vi "PTSequencer.dialog edit step.vi"(0 "Step List In":T4[](array[typedef]), 3 "i step":i32, 4 "new":bool, 5 "error in (no error)":errorcluster, 6 "read only":bool) -> (14 "Step List Out":T4[](array[typedef]), 16 "Step Out":T4, 18 "changed":bool, 19 "error out":errorcluster)   [LabVIEW 2014, in "PTSequencer.lvlib"]
uses:
  PTSequencer.lvlib
  _typedefs/method parameters/method parameters.xctl
  PTSequencer.step.ctl
  CSCore/CSSystem/CoreDefs/CoreDefs.rawDataType.ctl
  PTSequencer.DIM service condition.ctl
  _typedefs/X DIM conditions/X DIM conditions.xctl
  <vilib>/Utility/miscctls.llb/LVStringsAndValuesArrayTypeDef.ctl
  CSCore/CSSystem/CoreLib/CoreLib.byte array 2 string.vi
  CSCore/CSSystem/CoreLib/CoreLib.byte array 2 int.vi
  CSCore/CSSystem/CoreLib/CoreLib.byte array 2 int array.vi
  CSCore/CSSystem/CoreLib/CoreLib.byte array 2 short.vi
  CSCore/CSSystem/CoreLib/CoreLib.byte array 2 short array.vi
  CSCore/CSSystem/CoreLib/CoreLib.byte array 2 double.vi
  CSCore/CSSystem/CoreLib/CoreLib.byte array 2 double array.vi
  CSCore/CSSystem/CoreLib/CoreLib.byte array 2 float.vi
  CSCore/CSSystem/CoreLib/CoreLib.byte array 2 float array.vi
  _common/PTUtils/PTUtils.lvlib
  CSCore/CSSystem/CSSystemLib/CSSystemLib.lvlib
  CSCore/CSSystem/CoreLib/CoreLib.lvlib
panel:
  in  "Jump_failed":i32(ring) caption="if failed, jump to"
  in  "DIM Services ctl":T3
  in  "Delay":dbl caption="s"
  in  "delay":bool caption="use delay"
  out "Descriptors":string[](array[string])
  in  "DIM Services":T3(xcontrol) caption="DIM conditions"
  out "Errors":string
  in  "Step In":T4
  in  "Cancel":bool
  in  "Ok":bool
  out "subsequence":bool
  in  "Jump_passed":i32(ring) caption="if passed, jump to"
  in  "Failed":enum16{"Next", "Previous", "Repeat", "Jump"}(ring)
  in  "Passed":enum16{"Next", "Previous", "Repeat", "Jump"}(ring)
  in  "check":bool caption="use conditions"
  in  "Output Params":T5(xcontrol) caption="Output Parameters"
  in  "Input Params":T5(xcontrol) caption="Input Parameters"
  in  "Call Mode":enum16{"Simple DIM", "Synchronous"}(ring) caption="Call mode"
  in  "Method":u16(ring) items=["Ping", "GetDescriptors", "SetPdcInterval", "SetPdcPreset", "SetEvtPreset", "GetEvtStatus", "GetCNames", "GetIList", "Reset", "ReadData", "STOP", "Wait", "WakeupPeriodic", "GetVersionOfLibrary", "SetEvtPresetValue", "SetPdcPresetValue", "LoadProcess", "UnloadProcess", "RemoveAll", "ConnectProcess", "DisconnectProcess", "DisconnectAll", "GetClassNames", "GetObjectNames", "KillObject", "KillClass", "KillAllClasses", "SyncProcTable", "OpenFrontPanel", "RegisterProcess", "UnregisterProcess", "CreateObject", "DestroyObject"]
  in  "Object":u16(ring) items=["MainSystem\\Super", "MainSystem\\UserGOG", "MainSystem\\UserGOG_NotiObj", "OPCGatewayHV", "OPCGatewayLV", "PTScanner", "PT_CAEN_Gateway\\Super", "SimAFG"]
  in  "Description":string
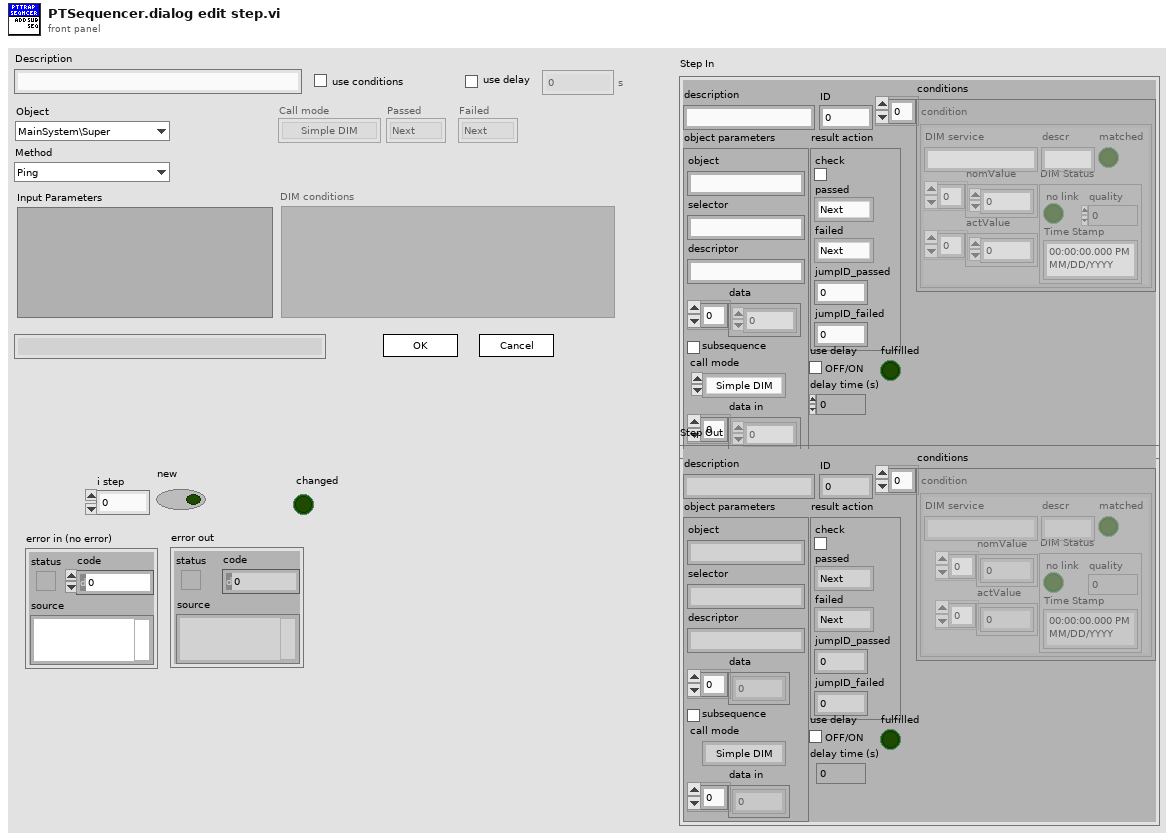
[diagram p1: front panel]
types:
  T1 = typedef "PTSequencer.lvlib/PTSequencer.DIM service condition.ctl" = cluster{"DIM service":string, "descr":string, "nomValue":T2, "actValue":T2, "matched":bool, "DIM Status":cluster{"no link":bool, "quality":i32, "Time Stamp":timestamp}}
  T2 = typedef "CoreDefs.rawDataType.ctl" = i8[]
  T3 = cluster{"DIM Services":string[], "data decsriptors":string[], "stop conditions":T1[]}
  T4 = typedef "PTSequencer.lvlib/PTSequencer.step.ctl" = cluster{"description":string, "object parameters":cluster{"object":string, "selector":string, "descriptor":string, "data":T2, "subsequence":bool, "call mode":enum16{"Simple DIM", "Synchronous"}, "data in":T2}, "result action":cluster{"check":bool, "passed":enum16{"Next", "Previous", "Repeat", "Jump"}, "failed":enum16{"Next", "Previous", "Repeat", "Jump"}, "jumpID_passed":i32, "jumpID_failed":i32}, "conditions":T1[], "fulfilled ":bool, "use delay":bool, "delay time (s)":dbl, "ID":i32}
  T5 = cluster{"Name":string, "Descr":string, "Value":string}[]
  T6 = enum8{"Enabled", "Disabled", "Disabled and Grayed Out"}
  T7 = typedef "LVStringsAndValuesArrayTypeDef.ctl" = cluster{"String":string, "Value":ext}[]
  T8 = cluster{"Name":string, "Descr":string, "Value":string}
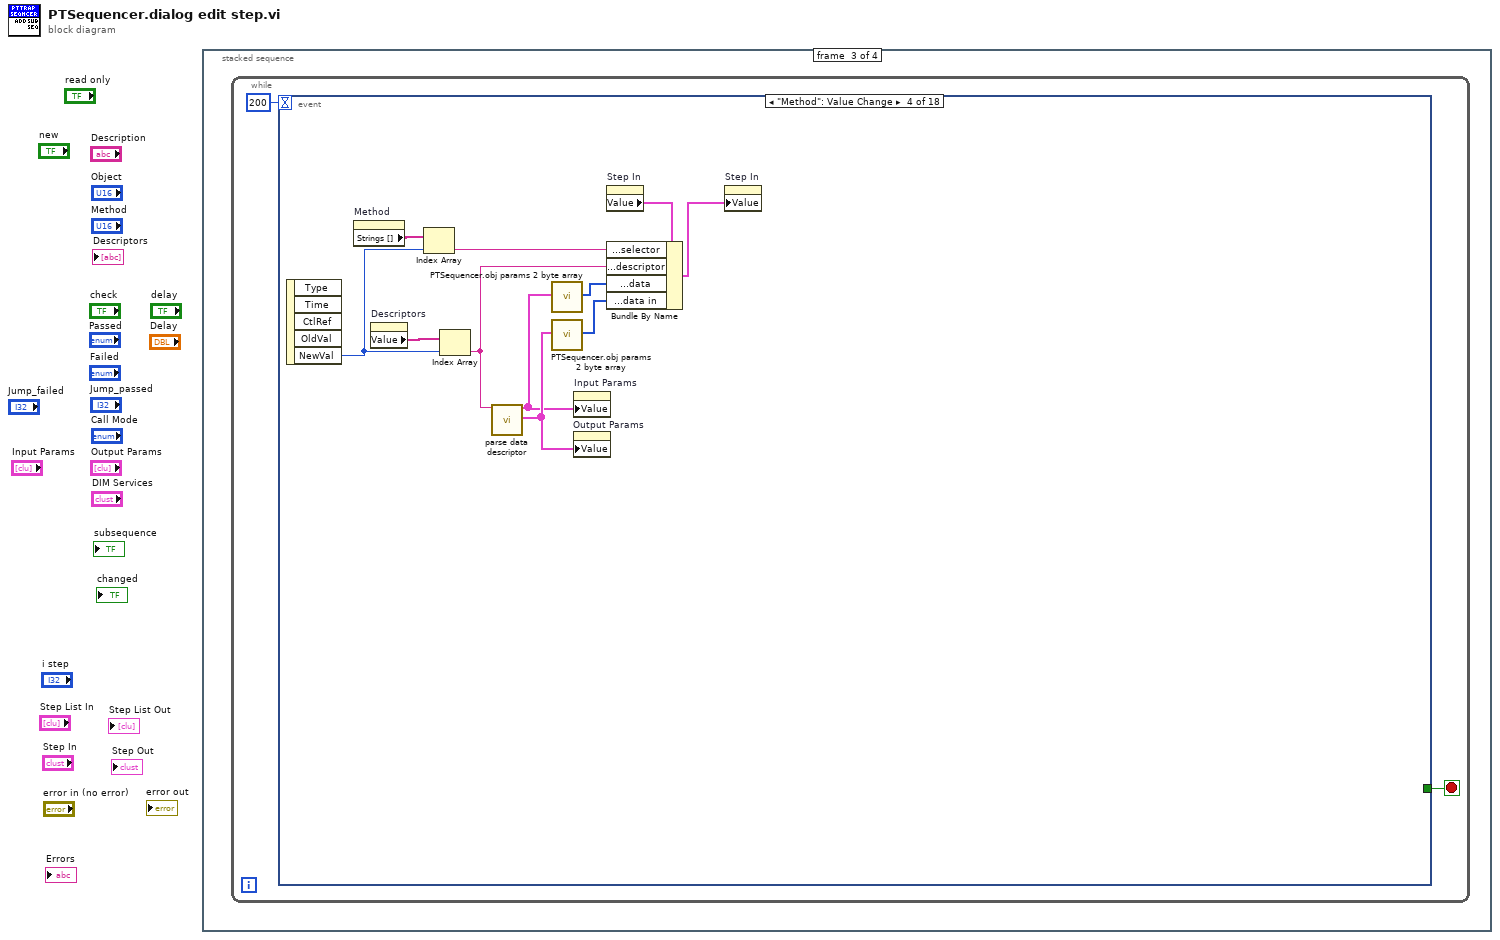
[diagram p0: block diagram]
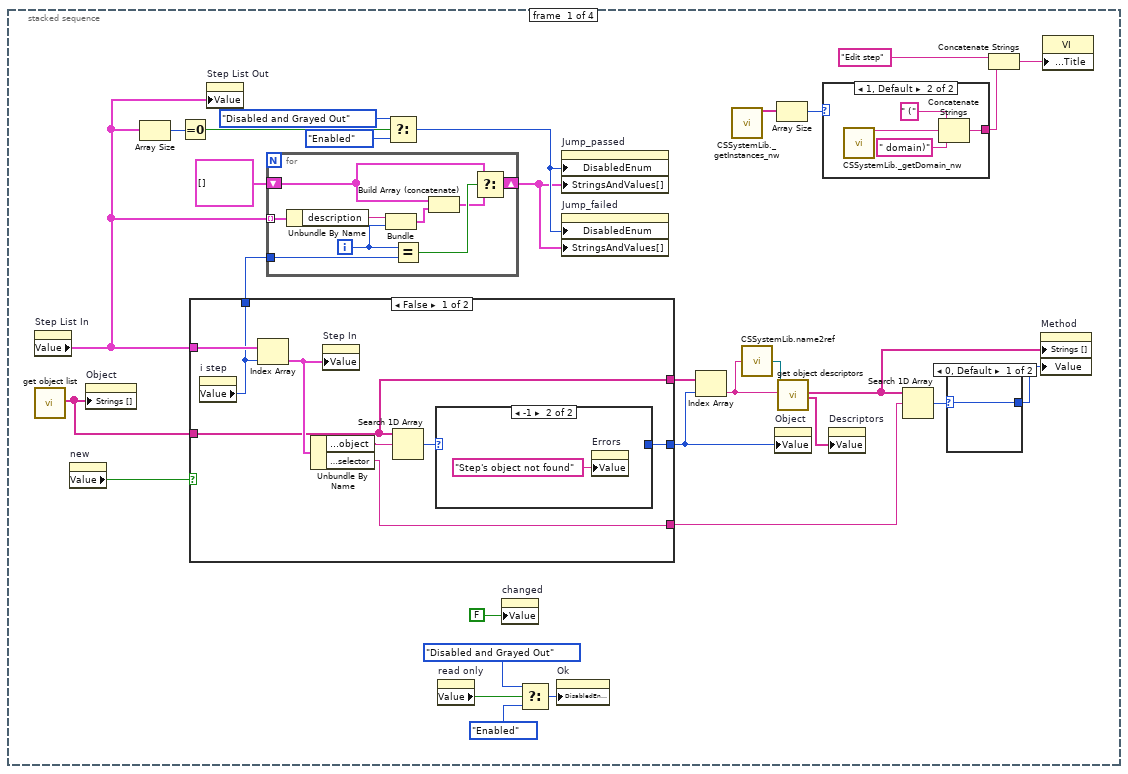
[diagram p2: hidden frame]
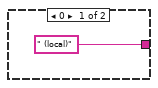
[diagram p3: hidden frame]
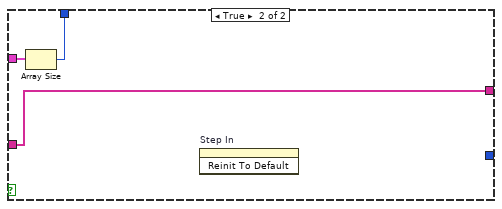
[diagram p6: hidden frame]
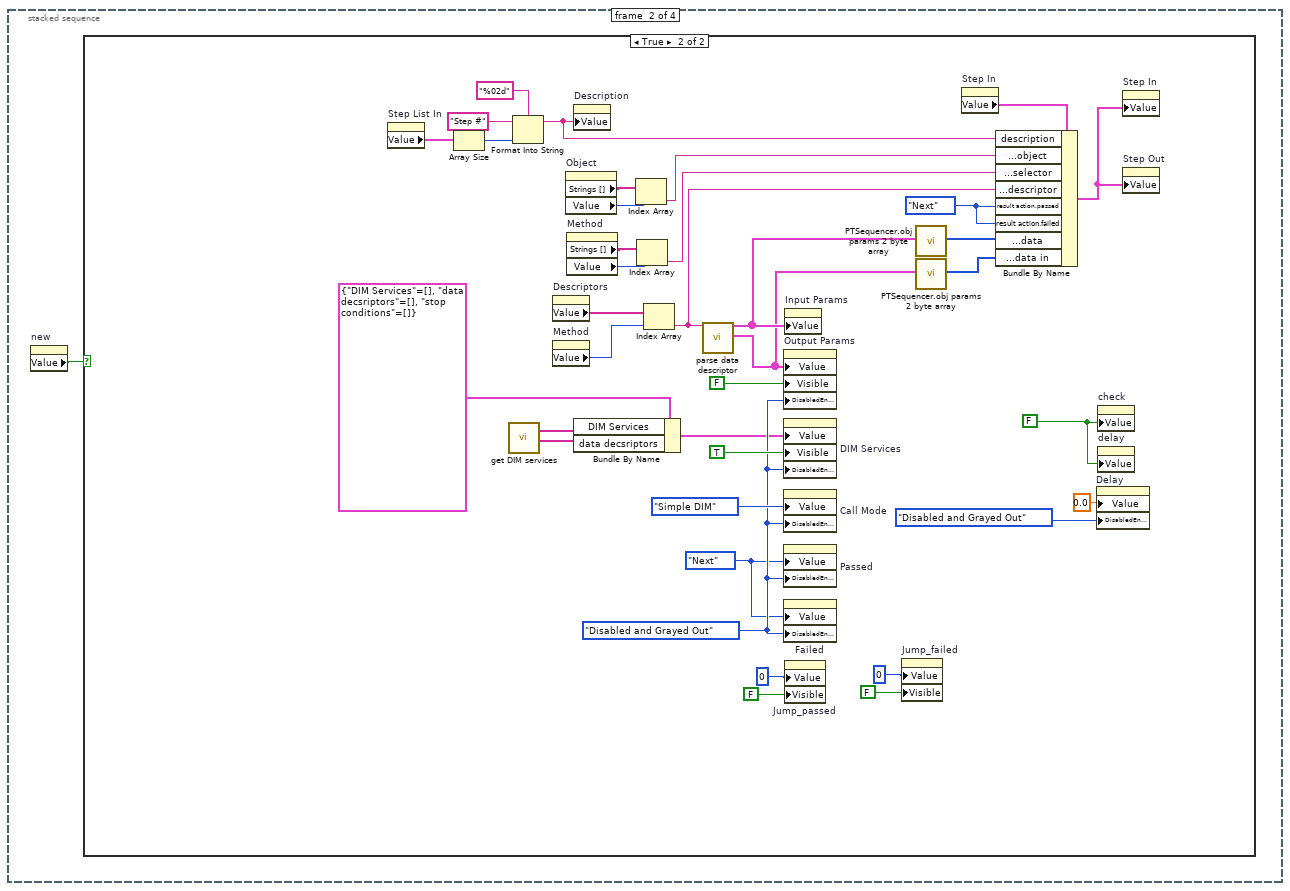
[diagram p7: hidden frame]
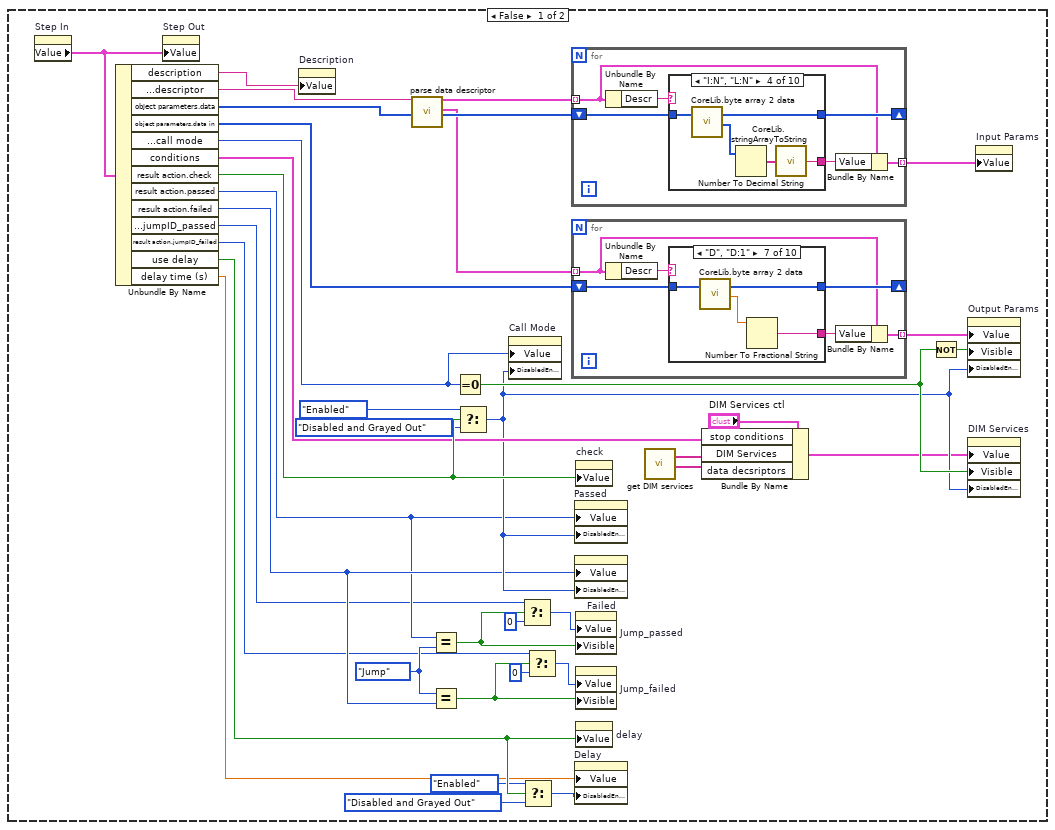
[diagram p8: hidden frame]
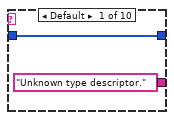
[diagram p9: hidden frame]
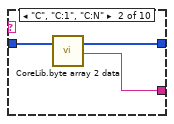
[diagram p10: hidden frame]
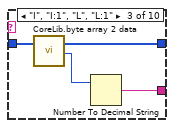
[diagram p11: hidden frame]
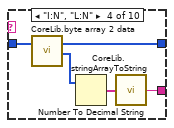
[diagram p12: hidden frame]
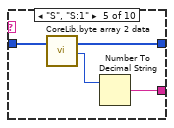
[diagram p13: hidden frame]
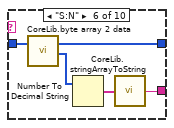
[diagram p14: hidden frame]
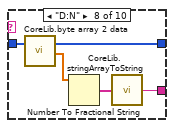
[diagram p15: hidden frame]
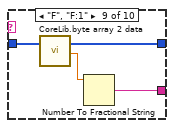
[diagram p16: hidden frame]
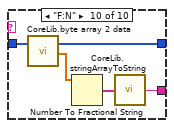
[diagram p17: hidden frame]
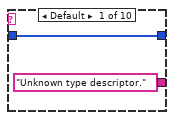
[diagram p18: hidden frame]
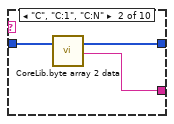
[diagram p19: hidden frame]
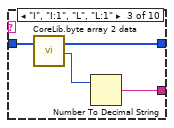
[diagram p20: hidden frame]
diagram:
  n1 = stacked-sequence {
    frame #0 {
      n2 = property on="Step List In" class="Arr (strict)"() -> ("Value"=w16:T4[])  [unwired: 2 in, 2 out]
      n3 = call "get object list.vi"() -> ("Objects"=w29:string[])  [unwired: 19 in]
      n4 = property on="new" class="Bool (strict)"() -> ("Value"=w30:bool)  [unwired: 2 in, 2 out]
      n5 = property on="Object" class="Ring (strict)"("Strings []"=w29) -> ()  [unwired: 2 in, 2 out]
      n6 = Array Size(array=w16) -> (size(s)=w15:i32)
      n7 = Equal To 0?(x=w15) -> (x = 0?=w14:bool)
      n8 = case shown="False" w30 {
        tunnel: w29 -> [w47 w58]
        tunnel: w16 -> [w50 w57]
        tunnel: [w49 w56] -> w27
        tunnel: [w48 _] -> w24
        tunnel: [w47 w58] -> w25
        tunnel: [w46 _] -> w22
        frame False {
          n9 = property on="i step" class="DigNum (strict)"() -> ("Value"=w49:i32)  [unwired: 2 in, 2 out]
          n10 = Index Array(array=w50, index=w49) -> (element=w53:T4)
          n11 = Unbundle By Name(w53) -> ("object parameters.object"=w52:string, "object parameters.selector"=w46:string)
          n12 = property on="Step In" class="Clust (strict)"("Value"=w53) -> ()  [unwired: 2 in, 2 out]
          n13 = Search 1D Array(1D array=w47, element=w52) -> (index of element=w51:i32)  [unwired: 1 in]
          n14 = case shown="-1" w51 {
            selector: w51 -> [w54 _]
            tunnel: [w54 _] -> w48
            frame 0, Default {
            }
            frame -1 {
              n15 = property on="Errors" class="Str"("Value"="Step's object not found") -> ()  [unwired: 2 in, 2 out]
            }
          }
        }
        frame True {
          n16 = Array Size(array=w57) -> (size(s)=w56:i32)
          n17 = invoke on="Step In" class="Clust (strict)" method="Reinit To Default"() -> ()  [unwired: 3 in, 3 out]
        }
      }
      n18 = property on="Step List Out" class="Arr (strict)"("Value"=w16) -> ()  [unwired: 2 in, 2 out]
      n19 = for {
        tunnel: w16 -> [w45] mode=indexing
        tunnel: w27 -> [w43]
        shift-right: [w37] -> w5
        shift-left: T7 [] ("Strings And Values []") -> [w38]
        i -> [w42]
        n20 = Unbundle By Name(w45) -> ("description"=w44:string)
        n21 = Bundle("description"=w44, w42) -> (w40:cluster{"description":string, i32})  [unwired: 1 in]
        n22 = Equal?(x=w42, y=w43) -> (x = y?=w41:bool)
        n23 = Build Array (concatenate)(w38, w40) -> (w39:T7)
        n24 = Select(t=w38, s=w41, f=w39) -> (s? t:f=w37:T7)
      }
      n25 = Select(t=T6."Disabled and Grayed Out" ("Disabled"), s=w14, f=T6."Enabled" ("Disabled")) -> (s? t:f=w6:T6)
      n26 = property on="read only" class="Bool (strict)"() -> ("Value"=w4:bool)  [unwired: 2 in, 2 out]
      n27 = property on="changed" class="Bool (strict)"("Value"=FALSE ("changed")) -> ()  [unwired: 2 in, 2 out]
      n28 = Select(t=T6."Disabled and Grayed Out" ("Disabled"), s=w4, f=T6."Enabled" ("Disabled")) -> (s? t:f=w3:T6)
      n29 = property on="Ok" class="Bool"("DisabledEnum"=w3) -> ()  [unwired: 2 in, 2 out]
      n30 = property on="Jump_passed" class="Ring (strict)"("DisabledEnum"=w6, "StringsAndValues[]"=w5) -> ()  [unwired: 2 in, 2 out]
      n31 = property on="Jump_failed" class="Ring (strict)"("DisabledEnum"=w6, "StringsAndValues[]"=w5) -> ()  [unwired: 2 in, 2 out]
      n32 = Index Array(array=w25, index=w24) -> (element=w23:string)
      n33 = call "CSSystemLib._getInstances_nw.vi"() -> ("i list"=w10:string[])  [unwired: 18 in, 1 out]
      n34 = call "CSSystemLib.name2ref.vi"("name"=w23) -> ("obj refnum"=w26:refnum<vi>)
      n35 = property on="Object" class="Ring (strict)"("Value"=w24) -> ()  [unwired: 2 in, 2 out]
      n36 = Array Size(array=w10) -> (size(s)=w11:i32)
      n37 = call "get object descriptors.vi"("i ref in"=w26, "Object"=w23) -> ("selectors"=w21:string[], "Descriptors"=w18:string[])  [unwired: 14 in, 2 out]
      n38 = case shown="1, Default" w11 {
        tunnel: [" (local)" w32] -> w8
        frame 0 {
        }
        frame 1, Default {
          n39 = call "CSSystemLib._getDomain_nw.vi"() -> ("CSDomain"=w34:string)  [unwired: 18 in, 1 out]
          n40 = Concatenate Strings(" (", w34, " domain)") -> (w32:string)
        }
      }
      n41 = property on="Descriptors" class="Arr (strict)"("Value"=w18) -> ()  [unwired: 2 in, 2 out]
      n42 = Search 1D Array(1D array=w21, element=w22) -> (index of element=w20:i32)  [unwired: 1 in]
      n43 = case shown="0, Default" w20 {
        selector: w20 -> [w36 _]
        tunnel: [w36 _] -> w19
        frame 0, Default {
        }
        frame -1 {
        }
      }
      n44 = Concatenate Strings("Edit step", w8) -> (w7:string)
      n45 = property on="Method" class="Ring (strict)"("Strings []"=w21, "Value"=w19) -> ()  [unwired: 2 in, 2 out]
      n46 = property class="VI"("Front Panel Window:Title"=w7) -> ()  [unwired: 2 in, 2 out]
    }
    frame #1 {
      n47 = property on="new" class="Bool (strict)"() -> ("Value"=w59:bool)  [unwired: 2 in, 2 out]
      n48 = case shown="True" w59 {
        frame False {
          w67 = enum16{"Next", "Previous", "Repeat", "Jump"}."Jump" ("y")
          n49 = property on="Step In" class="Clust (strict)"() -> ("Value"=w74:T4)  [unwired: 2 in, 2 out]
          n50 = Unbundle By Name(w74) -> ("description"=w68:string, "object parameters.descriptor"=w96:string, "object parameters.data"=w95:T2, "object parameters.data in"=w94:T2, "object parameters.call mode"=w93:enum16{"Simple DIM", "Synchronous"}, "conditions"=w83:T1[], "result action.check"=w92:bool, "result action.passed"=w66:enum16{"Next", "Previous", "Repeat", "Jump"}, "result action.failed"=w79:enum16{"Next", "Previous", "Repeat", "Jump"}, "result action.jumpID_passed"=w60:i32, "result action.jumpID_failed"=w61:i32, "use delay"=w73:bool, "delay time (s)"=w70:dbl)
          n51 = property on="Step Out" class="Clust (strict)"("Value"=w74) -> ()  [unwired: 2 in, 2 out]
          n52 = property on="Description" class="Str"("Value"=w68) -> ()  [unwired: 2 in, 2 out]
          n53 = call "parse data descriptor.vi"("dataDescriptor"=w96) -> ("Input Parameters"=w91:T5, "Output Parameters"=w89:T5)  [unwired: 14 in, 3 out]
          n54 = Equal?(x=w66, y=w67) -> (x = y?=w63:bool)
          n55 = Equal?(x=w67, y=w79) -> (x = y?=w64:bool)
          n56 = Equal To 0?(x=w93) -> (x = 0?=w87:bool)
          n57 = Select(t=T6."Enabled" ("Disabled"), s=w92, f=T6."Disabled and Grayed Out" ("Disabled")) -> (s? t:f=w80:T6)
          n58 = property on="Call Mode" class="Enum (strict)"("Value"=w93, "DisabledEnum"=w80) -> ()  [unwired: 2 in, 2 out]
          n59 = Select(t=w60, s=w63, f=0) -> (s? t:f=w62:i32)
          n60 = Select(t=T6."Enabled" ("Disabled"), s=w73, f=T6."Disabled and Grayed Out") -> (s? t:f=w69:T6)
          n61 = Select(t=w61, s=w64, f=0) -> (s? t:f=w76:i32)
          n62 = for {
            tunnel: w91 -> [w146] mode=indexing
            shift-right: [w147] -> _
            shift-left: w95 -> [w148]
            tunnel: [w144] -> w90 mode=indexing
            n63 = Unbundle By Name(w146) -> ("Descr"=w149:string)
            n64 = case shown="\"I:N\", \"L:N\"" w149 {
              tunnel: w148 -> [w151 w154 w158 w163 w167 w172 w176 w181 w184 w188]
              tunnel: [w151 w153 w157 w159 w164 w171 w175 w180 w182 w186] -> w147
              tunnel: ["Unknown type descriptor." w152 w155 w160 w165 w168 w173 w177 w183 w187] -> w145
              frame Default {
              }
              frame "C", "C:1", "C:N" {
                n65 = call-poly "CoreLib.byte array 2 data.vi"("byteArray"=w154) -> ("byteArray out"=w153:T2, "string"=w152:string)  [unwired: 16 in, 1 out]
              }
              frame "I", "I:1", "L", "L:1" {
                n66 = call-poly "CoreLib.byte array 2 data.vi"("byteArray"=w158) -> ("byteArray out"=w157:T2, "i32"=w156:i32)  [unwired: 16 in, 1 out]
                n67 = Number To Decimal String(number=w156) -> (decimal integer string=w155:string)  [unwired: 1 in]
              }
              frame "I:N", "L:N" {
                n68 = call-poly "CoreLib.byte array 2 data.vi"("byteArray"=w163) -> ("byteArray out"=w159:T2, "[i32]"=w162:i32[])  [unwired: 16 in, 1 out]
                n69 = Number To Decimal String(number=w162) -> (decimal integer string=w161:string[])  [unwired: 1 in]
                n70 = call "CoreLib.stringArrayToString.vi"("Array"=w161) -> ("String"=w160:string)
              }
              frame "S", "S:1" {
                n71 = call-poly "CoreLib.byte array 2 data.vi"("byteArray"=w167) -> ("byteArray out"=w164:T2, "i16"=w166:i16)  [unwired: 16 in, 1 out]
                n72 = Number To Decimal String(number=w166) -> (decimal integer string=w165:string)  [unwired: 1 in]
              }
              frame "S:N" {
                n73 = call-poly "CoreLib.byte array 2 data.vi"("byteArray"=w172) -> ("byteArray out"=w171:T2, "[i16]"=w170:i16[])  [unwired: 16 in, 1 out]
                n74 = Number To Decimal String(number=w170) -> (decimal integer string=w169:string[])  [unwired: 1 in]
                n75 = call "CoreLib.stringArrayToString.vi"("Array"=w169) -> ("String"=w168:string)
              }
              frame "D", "D:1" {
                n76 = call-poly "CoreLib.byte array 2 data.vi"("byteArray"=w176) -> ("byteArray out"=w175:T2, "d64"=w174:dbl)  [unwired: 16 in, 1 out]
                n77 = Number To Fractional String(number=w174) -> (F-format string=w173:string)  [unwired: 3 in]
              }
              frame "D:N" {
                n78 = call-poly "CoreLib.byte array 2 data.vi"("byteArray"=w181) -> ("byteArray out"=w180:T2, "[d64]"=w179:dbl[])  [unwired: 16 in, 1 out]
                n79 = Number To Fractional String(number=w179) -> (F-format string=w178:string[])  [unwired: 3 in]
                n80 = call "CoreLib.stringArrayToString.vi"("Array"=w178) -> ("String"=w177:string)
              }
              frame "F", "F:1" {
                n81 = call-poly "CoreLib.byte array 2 data.vi"("byteArray"=w184) -> ("byteArray out"=w182:T2, "f32"=w185:sgl)  [unwired: 16 in, 1 out]
                n82 = Number To Fractional String(number=w185) -> (F-format string=w183:string)  [unwired: 3 in]
              }
              frame "F:N" {
                n83 = call-poly "CoreLib.byte array 2 data.vi"("byteArray"=w188) -> ("byteArray out"=w186:T2, "[f32]"=w190:sgl[])  [unwired: 16 in, 1 out]
                n84 = Number To Fractional String(number=w190) -> (F-format string=w189:string[])  [unwired: 3 in]
                n85 = call "CoreLib.stringArrayToString.vi"("Array"=w189) -> ("String"=w187:string)
              }
            }
            n86 = Bundle By Name(cluster=w146, "Value"=w145) -> (w144:T8)
          }
          n87 = for {
            tunnel: w89 -> [w99] mode=indexing
            shift-right: [w100] -> _
            shift-left: w94 -> [w101]
            tunnel: [w97] -> w88 mode=indexing
            n88 = Unbundle By Name(w99) -> ("Descr"=w102:string)
            n89 = case shown="\"D\", \"D:1\"" w102 {
              tunnel: w101 -> [w104 w107 w111 w116 w120 w125 w129 w134 w137 w141]
              tunnel: [w104 w106 w110 w112 w117 w124 w128 w133 w135 w139] -> w100
              tunnel: ["Unknown type descriptor." w105 w108 w113 w118 w121 w126 w130 w136 w140] -> w98
              frame Default {
              }
              frame "C", "C:1", "C:N" {
                n90 = call-poly "CoreLib.byte array 2 data.vi"("byteArray"=w107) -> ("byteArray out"=w106:T2, "string"=w105:string)  [unwired: 16 in, 1 out]
              }
              frame "I", "I:1", "L", "L:1" {
                n91 = call-poly "CoreLib.byte array 2 data.vi"("byteArray"=w111) -> ("byteArray out"=w110:T2, "i32"=w109:i32)  [unwired: 16 in, 1 out]
                n92 = Number To Decimal String(number=w109) -> (decimal integer string=w108:string)  [unwired: 1 in]
              }
              frame "I:N", "L:N" {
                n93 = call-poly "CoreLib.byte array 2 data.vi"("byteArray"=w116) -> ("byteArray out"=w112:T2, "[i32]"=w115:i32[])  [unwired: 16 in, 1 out]
                n94 = Number To Decimal String(number=w115) -> (decimal integer string=w114:string[])  [unwired: 1 in]
                n95 = call "CoreLib.stringArrayToString.vi"("Array"=w114) -> ("String"=w113:string)
              }
              frame "S", "S:1" {
                n96 = call-poly "CoreLib.byte array 2 data.vi"("byteArray"=w120) -> ("byteArray out"=w117:T2, "i16"=w119:i16)  [unwired: 16 in, 1 out]
                n97 = Number To Decimal String(number=w119) -> (decimal integer string=w118:string)  [unwired: 1 in]
              }
              frame "S:N" {
                n98 = call-poly "CoreLib.byte array 2 data.vi"("byteArray"=w125) -> ("byteArray out"=w124:T2, "[i16]"=w123:i16[])  [unwired: 16 in, 1 out]
                n99 = Number To Decimal String(number=w123) -> (decimal integer string=w122:string[])  [unwired: 1 in]
                n100 = call "CoreLib.stringArrayToString.vi"("Array"=w122) -> ("String"=w121:string)
              }
              frame "D", "D:1" {
                n101 = call-poly "CoreLib.byte array 2 data.vi"("byteArray"=w129) -> ("byteArray out"=w128:T2, "d64"=w127:dbl)  [unwired: 16 in, 1 out]
                n102 = Number To Fractional String(number=w127) -> (F-format string=w126:string)  [unwired: 3 in]
              }
              frame "D:N" {
                n103 = call-poly "CoreLib.byte array 2 data.vi"("byteArray"=w134) -> ("byteArray out"=w133:T2, "[d64]"=w132:dbl[])  [unwired: 16 in, 1 out]
                n104 = Number To Fractional String(number=w132) -> (F-format string=w131:string[])  [unwired: 3 in]
                n105 = call "CoreLib.stringArrayToString.vi"("Array"=w131) -> ("String"=w130:string)
              }
              frame "F", "F:1" {
                n106 = call-poly "CoreLib.byte array 2 data.vi"("byteArray"=w137) -> ("byteArray out"=w135:T2, "f32"=w138:sgl)  [unwired: 16 in, 1 out]
                n107 = Number To Fractional String(number=w138) -> (F-format string=w136:string)  [unwired: 3 in]
              }
              frame "F:N" {
                n108 = call-poly "CoreLib.byte array 2 data.vi"("byteArray"=w141) -> ("byteArray out"=w139:T2, "[f32]"=w143:sgl[])  [unwired: 16 in, 1 out]
                n109 = Number To Fractional String(number=w143) -> (F-format string=w142:string[])  [unwired: 3 in]
                n110 = call "CoreLib.stringArrayToString.vi"("Array"=w142) -> ("String"=w140:string)
              }
            }
            n111 = Bundle By Name(cluster=w99, "Value"=w98) -> (w97:T8)
          }
          n112 = property on="Passed" class="Enum (strict)"("Value"=w66, "DisabledEnum"=w80) -> ()  [unwired: 2 in, 2 out]
          n113 = property on="Failed" class="Enum (strict)"("Value"=w79, "DisabledEnum"=w80) -> ()  [unwired: 2 in, 2 out]
          n114 = property on="Delay" class="DigNum (strict)"("Value"=w70, "DisabledEnum"=w69) -> ()  [unwired: 2 in, 2 out]
          n115 = property on="check" class="Bool (strict)"("Value"=w92) -> ()  [unwired: 2 in, 2 out]
          n116 = property on="Jump_passed" class="Ring (strict)"("Value"=w62, "Visible"=w63) -> ()  [unwired: 2 in, 2 out]
          n117 = property on="Jump_failed" class="Ring (strict)"("Value"=w76, "Visible"=w64) -> ()  [unwired: 2 in, 2 out]
          n118 = property on="delay" class="Bool (strict)"("Value"=w73) -> ()  [unwired: 2 in, 2 out]
          n119 = call "get DIM services.vi"() -> ("services"=w82:string[], "descriptors"=w81:string[])  [unwired: 17 in, 1 out]
          n120 = Bundle By Name(cluster="DIM Services ctl", "stop conditions"=w83, "DIM Services"=w82, "data decsriptors"=w81) -> (w77:T3)
          n121 = Not(x=w87) -> (.not. x?=w86:bool)
          n122 = property on="Output Params" class="method parameters (strict)"("Value"=w88, "Visible"=w86, "DisabledEnum"=w80) -> ()  [unwired: 2 in, 2 out]
          n123 = property on="DIM Services" class="X DIM conditions (strict)"("Value"=w77, "Visible"=w87, "DisabledEnum"=w80) -> ()  [unwired: 2 in, 2 out]
          n124 = property on="Input Params" class="method parameters (strict)"("Value"=w90) -> ()  [unwired: 2 in, 2 out]
        }
        frame True {
          w192 = enum16{"Next", "Previous", "Repeat", "Jump"}."Next" ("result action.passed")
          w191 = enum16{"Next", "Previous", "Repeat", "Jump"}."Next"
          w202 = FALSE
          w220 = T6."Disabled and Grayed Out" ("Disabled")
          n125 = property on="Step List In" class="Arr (strict)"() -> ("Value"=w227:T4[])  [unwired: 2 in, 2 out]
          n126 = Array Size(array=w227) -> (size(s)=w226:i32)
          n127 = call "get DIM services.vi"() -> ("services"=w219:string[], "descriptors"=w218:string[])  [unwired: 17 in, 1 out]
          n128 = Format Into String(format string="%02d", initial string="Step #", w226) -> (resulting string=w200:string)  [unwired: 1 in, 1 out]
          n129 = property on="Descriptors" class="Arr (strict)"() -> ("Value"=w217:string[])  [unwired: 2 in, 2 out]
          n130 = property on="Method" class="Ring (strict)"() -> ("Value"=w216:u16)  [unwired: 2 in, 2 out]
          n131 = property on="Object" class="Ring (strict)"() -> ("Strings []"=w214:string[], "Value"=w213:u16)  [unwired: 2 in, 2 out]
          n132 = property on="Method" class="Ring (strict)"() -> ("Strings []"=w210:string[], "Value"=w211:u16)  [unwired: 2 in, 2 out]
          n133 = property on="Description" class="Str"("Value"=w200) -> ()  [unwired: 2 in, 2 out]
          n134 = Bundle By Name(cluster=T3 {"DIM Services"=[], "data decsriptors"=[], "stop conditions"=[]} ("DIM Services ctl"), "DIM Services"=w219, "data decsriptors"=w218) -> (w205:T3)
          n135 = Index Array(array=w214, index=w213) -> (element=w212:string)
          n136 = Index Array(array=w210, index=w211) -> (element=w209:string)
          n137 = Index Array(array=w217, index=w216) -> (element=w207:string)
          n138 = call "parse data descriptor.vi"("dataDescriptor"=w207) -> ("Input Parameters"=w198:T5, "Output Parameters"=w197:T5)  [unwired: 14 in, 3 out]
          n139 = property on="Output Params" class="method parameters (strict)"("Value"=w197, "Visible"=FALSE, "DisabledEnum"=w220) -> ()  [unwired: 2 in, 2 out]
          n140 = property on="DIM Services" class="X DIM conditions (strict)"("Value"=w205, "Visible"=TRUE, "DisabledEnum"=w220) -> ()  [unwired: 2 in, 2 out]
          n141 = property on="Call Mode" class="Enum (strict)"("Value"=enum16{"Simple DIM", "Synchronous"}."Simple DIM" ("object parameters.call mode"), "DisabledEnum"=w220) -> ()  [unwired: 2 in, 2 out]
          n142 = property on="Passed" class="Enum (strict)"("Value"=w191, "DisabledEnum"=w220) -> ()  [unwired: 2 in, 2 out]
          n143 = property on="Failed" class="Enum (strict)"("Value"=w191, "DisabledEnum"=w220) -> ()  [unwired: 2 in, 2 out]
          n144 = property on="Input Params" class="method parameters (strict)"("Value"=w198) -> ()  [unwired: 2 in, 2 out]
          n145 = property on="Jump_passed" class="Ring (strict)"("Value"=0, "Visible"=FALSE) -> ()  [unwired: 2 in, 2 out]
          n146 = property on="Jump_failed" class="Ring (strict)"("Value"=0, "Visible"=FALSE) -> ()  [unwired: 2 in, 2 out]
          n147 = call "PTSequencer.obj params 2 byte array.vi"("method parameters"=w198) -> ("byteArray out"=w196:T2)  [unwired: 18 in]
          n148 = call "PTSequencer.obj params 2 byte array.vi"("method parameters"=w197) -> ("byteArray out"=w195:T2)  [unwired: 18 in]
          n149 = property on="Step In" class="Clust (strict)"() -> ("Value"=w215:T4)  [unwired: 2 in, 2 out]
          n150 = Bundle By Name(cluster=w215, "description"=w200, "object parameters.object"=w212, "object parameters.selector"=w209, "object parameters.descriptor"=w207, "result action.passed"=w192, "result action.failed"=w192, "object parameters.data"=w196, "object parameters.data in"=w195) -> (w204:T4)
          n151 = property on="Delay" class="DigNum (strict)"("Value"=0.0 ("Delay"), "DisabledEnum"=T6."Disabled and Grayed Out" ("f")) -> ()  [unwired: 2 in, 2 out]
          n152 = property on="check" class="Bool (strict)"("Value"=w202) -> ()  [unwired: 2 in, 2 out]
          n153 = property on="delay" class="Bool (strict)"("Value"=w202) -> ()  [unwired: 2 in, 2 out]
          n154 = property on="Step In" class="Clust (strict)"("Value"=w204) -> ()  [unwired: 2 in, 2 out]
          n155 = property on="Step Out" class="Clust (strict)"("Value"=w204) -> ()  [unwired: 2 in, 2 out]
        }
      }
    }
    frame #2 {
      n156 = while {
        stop <- w229 stop-if-true
        n157 = event shown="[3] \"Method\": Value Change" {
          selector: _ -> [_ _ _ _ _ _ _ _ _ _ _ _ _ _ _ _ _ _]
          dyn-events: _ -> [_ _ _ _ _ _ _ _ _ _ _ _ _ _ _ _ _ _]
          timeout: 200 -> [_ _ _ _ _ _ _ _ _ _ _ _ _ _ _ _ _ _]
          tunnel: [_ _ _ _ _ _ _ _ _ _ _ _ _ _ _ TRUE TRUE w341] -> w229
          event Timeout {
            n158 = event-data() -> ()  [unwired: 1 in, 2 out]
          }
          event "Description": Value Change {
            n159 = event-data() -> ("NewVal"=w231:string)  [unwired: 1 in, 4 out]
            n160 = property on="Step In" class="Clust (strict)"() -> ("Value"=w232:T4)  [unwired: 2 in, 2 out]
            n161 = Bundle By Name(cluster=w232, "description"=w231) -> (w230:T4)
            n162 = property on="Step In" class="Clust (strict)"("Value"=w230) -> ()  [unwired: 2 in, 2 out]
          }
          event "Object": Value Change {
            w239 = 0
            n163 = event-data() -> ("NewVal"=w243:u16)  [unwired: 1 in, 4 out]
            n164 = property on="Object" class="Ring (strict)"() -> ("Strings []"=w245:string[])  [unwired: 2 in, 2 out]
            n165 = Index Array(array=w245, index=w243) -> (element=w242:string)
            n166 = call "CSSystemLib.name2ref.vi"("name"=w242) -> ("obj refnum"=w244:refnum<vi>)
            n167 = call "get object descriptors.vi"("i ref in"=w244, "Object"=w242) -> ("selectors"=w240:string[], "Descriptors"=w241:string[])  [unwired: 14 in, 2 out]
            n168 = property on="Descriptors" class="Arr (strict)"("Value"=w241) -> ()  [unwired: 2 in, 2 out]
            n169 = property on="Method" class="Ring (strict)"("Strings []"=w240, "Value"=w239) -> ()  [unwired: 2 in, 2 out]
            n170 = Index Array(array=w240, index=w239) -> (element=w238:string)
            n171 = Index Array(array=w241, index=w239) -> (element=w237:string)
            n172 = call "parse data descriptor.vi"("dataDescriptor"=w237) -> ("Input Parameters"=w236:T5, "Output Parameters"=w235:T5)  [unwired: 14 in, 3 out]
            n173 = call "PTSequencer.obj params 2 byte array.vi"("method parameters"=w236) -> ("byteArray out"=w234:T2)  [unwired: 18 in]
            n174 = call "PTSequencer.obj params 2 byte array.vi"("method parameters"=w235) -> ("byteArray out"=w233:T2)  [unwired: 18 in]
            n175 = property on="Input Params" class="method parameters (strict)"("Value"=w236) -> ()  [unwired: 2 in, 2 out]
            n176 = property on="Output Params" class="method parameters (strict)"("Value"=w235) -> ()  [unwired: 2 in, 2 out]
            n177 = property on="Step In" class="Clust (strict)"() -> ("Value"=w247:T4)  [unwired: 2 in, 2 out]
            n178 = Bundle By Name(cluster=w247, "object parameters.object"=w242, "object parameters.selector"=w238, "object parameters.descriptor"=w237, "object parameters.data"=w234, "object parameters.data in"=w233) -> (w246:T4)
            n179 = property on="Step In" class="Clust (strict)"("Value"=w246) -> ()  [unwired: 2 in, 2 out]
          }
          event "Method": Value Change {
            n180 = event-data() -> ("NewVal"=w256:u16)  [unwired: 1 in, 4 out]
            n181 = property on="Method" class="Ring (strict)"() -> ("Strings []"=w257:string[])  [unwired: 2 in, 2 out]
            n182 = property on="Descriptors" class="Arr (strict)"() -> ("Value"=w258:string[])  [unwired: 2 in, 2 out]
            n183 = Index Array(array=w257, index=w256) -> (element=w253:string)
            n184 = Index Array(array=w258, index=w256) -> (element=w252:string)
            n185 = call "parse data descriptor.vi"("dataDescriptor"=w252) -> ("Input Parameters"=w250:T5, "Output Parameters"=w251:T5)  [unwired: 14 in, 3 out]
            n186 = call "PTSequencer.obj params 2 byte array.vi"("method parameters"=w250) -> ("byteArray out"=w249:T2)  [unwired: 18 in]
            n187 = call "PTSequencer.obj params 2 byte array.vi"("method parameters"=w251) -> ("byteArray out"=w248:T2)  [unwired: 18 in]
            n188 = property on="Input Params" class="method parameters (strict)"("Value"=w250) -> ()  [unwired: 2 in, 2 out]
            n189 = property on="Output Params" class="method parameters (strict)"("Value"=w251) -> ()  [unwired: 2 in, 2 out]
            n190 = property on="Step In" class="Clust (strict)"() -> ("Value"=w255:T4)  [unwired: 2 in, 2 out]
            n191 = Bundle By Name(cluster=w255, "object parameters.selector"=w253, "object parameters.descriptor"=w252, "object parameters.data"=w249, "object parameters.data in"=w248) -> (w254:T4)
            n192 = property on="Step In" class="Clust (strict)"("Value"=w254) -> ()  [unwired: 2 in, 2 out]
          }
          event "check": Value Change {
            n193 = event-data() -> ("NewVal"=w262:bool)  [unwired: 1 in, 4 out]
            n194 = property on="Step List In" class="Arr (strict)"() -> ("Value"=w264:T4[])  [unwired: 2 in, 2 out]
            n195 = Select(t=T6."Enabled" ("Disabled"), s=w262, f=T6."Disabled and Grayed Out" ("Disabled")) -> (s? t:f=w260:T6)
            n196 = property on="Step In" class="Clust (strict)"() -> ("Value"=w266:T4)  [unwired: 2 in, 2 out]
            n197 = Bundle By Name(cluster=w266, "result action.check"=w262) -> (w267:T4)
            n198 = Array Size(array=w264) -> (size(s)=w265:i32)
            n199 = Not Equal To 0?(x=w265) -> (x != 0?=w263:bool)
            n200 = property on="Step In" class="Clust (strict)"("Value"=w267) -> ()  [unwired: 2 in, 2 out]
            n201 = Select(t=w260, s=w263, f=T6."Disabled and Grayed Out" ("Disabled")) -> (s? t:f=w259:T6)
            n202 = property on="Output Params" class="method parameters (strict)"("DisabledEnum"=w260) -> ()  [unwired: 2 in, 2 out]
            n203 = property on="DIM Services" class="X DIM conditions (strict)"("DisabledEnum"=w260) -> ()  [unwired: 2 in, 2 out]
            n204 = property on="Call Mode" class="Enum (strict)"("DisabledEnum"=w260) -> ()  [unwired: 2 in, 2 out]
            n205 = property on="Passed" class="Enum (strict)"("DisabledEnum"=w260) -> ()  [unwired: 2 in, 2 out]
            n206 = property on="Failed" class="Enum (strict)"("DisabledEnum"=w260) -> ()  [unwired: 2 in, 2 out]
            n207 = property on="Jump_passed" class="Ring (strict)"("DisabledEnum"=w259) -> ()  [unwired: 2 in, 2 out]
            n208 = property on="Jump_failed" class="Ring (strict)"("DisabledEnum"=w259) -> ()  [unwired: 2 in, 2 out]
          }
          event "Passed": Value Change {
            n209 = event-data() -> ("NewVal"=w272:enum16{"Next", "Previous", "Repeat", "Jump"})  [unwired: 1 in, 4 out]
            n210 = property on="Step In" class="Clust (strict)"() -> ("Value"=w273:T4)  [unwired: 2 in, 2 out]
            n211 = Bundle By Name(cluster=w273, "result action.passed"=w272) -> (w274:T4)
            n212 = Equal?(x=w272, y=enum16{"Next", "Previous", "Repeat", "Jump"}."Jump") -> (x = y?=w270:bool)
            n213 = property on="Jump_passed" class="Ring (strict)"("Visible"=w270) -> ()  [unwired: 2 in, 2 out]
            n214 = property on="Step In" class="Clust (strict)"("Value"=w274) -> ()  [unwired: 2 in, 2 out]
          }
          event "Failed": Value Change {
            n215 = event-data() -> ("NewVal"=w277:enum16{"Next", "Previous", "Repeat", "Jump"})  [unwired: 1 in, 4 out]
            n216 = property on="Step In" class="Clust (strict)"() -> ("Value"=w278:T4)  [unwired: 2 in, 2 out]
            n217 = Bundle By Name(cluster=w278, "result action.failed"=w277) -> (w279:T4)
            n218 = Equal?(x=w277, y=enum16{"Next", "Previous", "Repeat", "Jump"}."Jump") -> (x = y?=w276:bool)
            n219 = property on="Jump_failed" class="Ring (strict)"("Visible"=w276) -> ()  [unwired: 2 in, 2 out]
            n220 = property on="Step In" class="Clust (strict)"("Value"=w279) -> ()  [unwired: 2 in, 2 out]
          }
          event "Jump_passed": Value Change {
            n221 = event-data() -> ("NewVal"=w280:i32)  [unwired: 1 in, 4 out]
            n222 = property on="Step In" class="Clust (strict)"() -> ("Value"=w281:T4)  [unwired: 2 in, 2 out]
            n223 = Bundle By Name(cluster=w281, "result action.jumpID_passed"=w280) -> (w282:T4)
            n224 = property on="Step In" class="Clust (strict)"("Value"=w282) -> ()  [unwired: 2 in, 2 out]
          }
          event "Jump_failed": Value Change {
            n225 = event-data() -> ("NewVal"=w283:i32)  [unwired: 1 in, 4 out]
            n226 = property on="Step In" class="Clust (strict)"() -> ("Value"=w284:T4)  [unwired: 2 in, 2 out]
            n227 = Bundle By Name(cluster=w284, "result action.jumpID_failed"=w283) -> (w285:T4)
            n228 = property on="Step In" class="Clust (strict)"("Value"=w285) -> ()  [unwired: 2 in, 2 out]
          }
          event "Call Mode": Value Change {
            n229 = event-data() -> ("NewVal"=w286:enum16{"Simple DIM", "Synchronous"})  [unwired: 1 in, 4 out]
            n230 = Equal To 0?(x=w286) -> (x = 0?=w290:bool)
            n231 = property on="Step In" class="Clust (strict)"() -> ("Value"=w288:T4)  [unwired: 2 in, 2 out]
            n232 = Bundle By Name(cluster=w288, "object parameters.call mode"=w286) -> (w287:T4)
            n233 = Not(x=w290) -> (.not. x?=w289:bool)
            n234 = property on="DIM Services" class="X DIM conditions (strict)"("Visible"=w290) -> ()  [unwired: 2 in, 2 out]
            n235 = property on="Output Params" class="method parameters (strict)"("Visible"=w289) -> ()  [unwired: 2 in, 2 out]
            n236 = property on="Step In" class="Clust (strict)"("Value"=w287) -> ()  [unwired: 2 in, 2 out]
          }
          event "delay": Value Change {
            n237 = event-data() -> ("NewVal"=w292:bool)  [unwired: 1 in, 4 out]
            n238 = Select(t=T6."Enabled" ("Disabled"), s=w292, f=T6."Disabled and Grayed Out" ("Disabled")) -> (s? t:f=w291:T6)
            n239 = property on="Step In" class="Clust (strict)"() -> ("Value"=w295:T4)  [unwired: 2 in, 2 out]
            n240 = Bundle By Name(cluster=w295, "use delay"=w292) -> (w296:T4)
            n241 = property on="Delay" class="DigNum (strict)"("DisabledEnum"=w291) -> ()  [unwired: 2 in, 2 out]
            n242 = property on="Step In" class="Clust (strict)"("Value"=w296) -> ()  [unwired: 2 in, 2 out]
          }
          event "Delay": Value Change {
            n243 = event-data() -> ("NewVal"=w297:dbl)  [unwired: 1 in, 4 out]
            n244 = property on="Step In" class="Clust (strict)"() -> ("Value"=w298:T4)  [unwired: 2 in, 2 out]
            n245 = Bundle By Name(cluster=w298, "delay time (s)"=w297) -> (w299:T4)
            n246 = property on="Step In" class="Clust (strict)"("Value"=w299) -> ()  [unwired: 2 in, 2 out]
          }
          event "Input Params": Value Change {
            n247 = event-data() -> ("NewVal"=w301:T5)  [unwired: 1 in, 4 out]
            n248 = call "PTSequencer.obj params 2 byte array.vi"("method parameters"=w301) -> ("byteArray out"=w300:T2)  [unwired: 18 in]
            n249 = property on="Step In" class="Clust (strict)"() -> ("Value"=w302:T4)  [unwired: 2 in, 2 out]
            n250 = Bundle By Name(cluster=w302, "object parameters.data"=w300) -> (w303:T4)
            n251 = property on="Step In" class="Clust (strict)"("Value"=w303) -> ()  [unwired: 2 in, 2 out]
          }
          event "Output Params": Value Change {
            n252 = event-data() -> ("NewVal"=w305:T5)  [unwired: 1 in, 4 out]
            n253 = call "PTSequencer.obj params 2 byte array.vi"("method parameters"=w305) -> ("byteArray out"=w304:T2)  [unwired: 18 in]
            n254 = property on="Step In" class="Clust (strict)"() -> ("Value"=w306:T4)  [unwired: 2 in, 2 out]
            n255 = Bundle By Name(cluster=w306, "object parameters.data in"=w304) -> (w307:T4)
            n256 = property on="Step In" class="Clust (strict)"("Value"=w307) -> ()  [unwired: 2 in, 2 out]
          }
          event "DIM Services": Value Change {
            n257 = event-data() -> ("NewVal"=w309:T3)  [unwired: 1 in, 4 out]
            n258 = Unbundle By Name(w309) -> ("stop conditions"=w308:T1[])
            n259 = property on="Step In" class="Clust (strict)"() -> ("Value"=w310:T4)  [unwired: 2 in, 2 out]
            n260 = Bundle By Name(cluster=w310, "conditions"=w308) -> (w311:T4)
            n261 = property on="Step In" class="Clust (strict)"("Value"=w311) -> ()  [unwired: 2 in, 2 out]
          }
          event "Ok": Value Change {
            n262 = event-data() -> ()  [unwired: 1 in, 5 out]
            n263 = property on="Call Mode" class="Enum (strict)"() -> ("Value"=w322:enum16{"Simple DIM", "Synchronous"})  [unwired: 2 in, 2 out]
            n264 = property on="check" class="Bool (strict)"() -> ("Value"=w323:bool)  [unwired: 2 in, 2 out]
            n265 = case shown="True" w323 {
              tunnel: w322 -> [_ w335]
              tunnel: [enum16{"Simple DIM", "Synchronous"}."Simple DIM" ("f") w333] -> w321
              tunnel: [_ w334] -> w320
              frame False {
              }
              frame True {
                n266 = case shown="\"Simple DIM\", Default" w335 {
                  selector: w335 -> [w336 w339]
                  tunnel: [w337 _] -> w334
                  tunnel: [w336 w339] -> w333
                  frame "Simple DIM", Default {
                    n267 = property on="DIM Services" class="X DIM conditions (strict)"() -> ("Value"=w338:T3)  [unwired: 2 in, 2 out]
                    n268 = Unbundle By Name(w338) -> ("stop conditions"=w337:T1[])
                  }
                  frame "Synchronous" {
                  }
                }
              }
            }
            n269 = property on="Step Out" class="Clust (strict)"() -> ("Value"=w315:T4)  [unwired: 2 in, 2 out]
            n270 = property on="Step In" class="Clust (strict)"() -> ("Value"=w316:T4)  [unwired: 2 in, 2 out]
            n271 = Bundle By Name(cluster=w316, "conditions"=w320, "object parameters.call mode"=w321) -> (w317:T4)
            n272 = property on="new" class="Bool (strict)"() -> ("Value"=w313:bool)  [unwired: 2 in, 2 out]
            n273 = Not Equal?(x=w315, y=w316) -> (x != y?=w312:bool)
            n274 = property on="Step Out" class="Clust (strict)"("Value"=w317) -> ()  [unwired: 2 in, 2 out]
            n275 = Or(x=w313, y=w312) -> (x .or. y?=w314:bool)
            n276 = property on="Step List In" class="Arr (strict)"() -> ("Value"=w319:T4[])  [unwired: 2 in, 2 out]
            n277 = property on="changed" class="Bool (strict)"("Value"=w314) -> ()  [unwired: 2 in, 2 out]
            n278 = case shown="False" w313 {
              tunnel: w319 -> [w328 w331]
              tunnel: [w326 w330] -> w318
              tunnel: w317 -> [w325 w329]
              frame False {
                n279 = property on="i step" class="DigNum (strict)"() -> ("Value"=w327:i32)  [unwired: 2 in, 2 out]
                n280 = Replace Array Subset(array=w328, new element=w325, index=w327) -> (w326:T4[])
              }
              frame True {
                n281 = Build Array (concatenate)(w331, w329) -> (w330:T4[])
              }
            }
            n282 = property on="Step List Out" class="Arr (strict)"("Value"=w318) -> ()  [unwired: 2 in, 2 out]
          }
          event "Cancel": Value Change {
            n283 = event-data() -> ()  [unwired: 1 in, 5 out]
          }
          event Panel Close? {
            w341 = TRUE
            n284 = event-data() -> ()  [unwired: 1 in, 3 out]
            n285 = event-data("Discard?"=w341) -> ()  [unwired: 1 in, 1 out]
          }
        }
      }
    }
    frame #3 {
      n286 = invoke class="VI" method="FP.Close"() -> ()  [unwired: 3 in, 3 out]
    }
  }
